vi "sync stream channels.vi"(7 "stream":T1 format="%.0x", 8 "error in":errorcluster, 10 "names":string[](array[string]), 11 "channels":T1[](array[typedef]) format="%.0x") -> (0 "error out":errorcluster, 2 "saved names":string[](array[string]), 3 "saved channels":T1[](array[typedef]) format="%.0x")   [LabVIEW 2026, in "Nominal Core Streaming System Explorer.lvlib"]
uses:
  Nominal Core Streaming System Explorer.lvlib
  <vilib>/NI VeriStand/Custom Device API/Custom Device Item Ref.ctl
  <vilib>/NI VeriStand/Custom Device API/Set Item Property (String Array).vi
  <vilib>/NI VeriStand/Custom Device API/Custom Device API.lvlib
  <vilib>/NI VeriStand/Custom Device Tools/Custom Device Utility Library/Custom Device Utility Library.lvlib
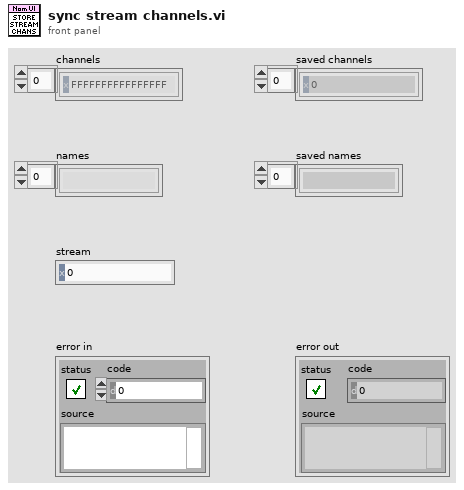
[diagram p1: front panel]
types:
  T1 = typedef "Custom Device API.lvlib/Custom Device Item Ref.ctl" = u64
  T2 = typedef "Custom Device API.lvlib/Custom Device Item Info.ctl" = cluster{"Name":string, "Is Channel":bool, "GUID":string, "Is Waveform":bool}
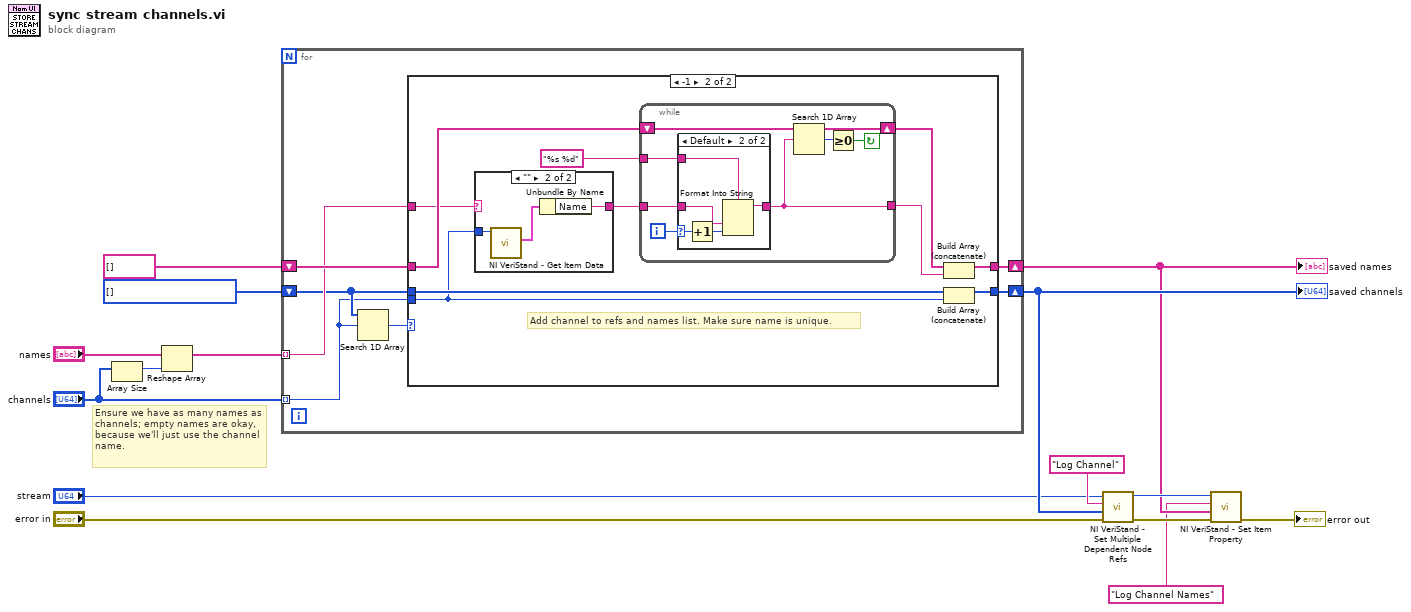
[diagram p0: block diagram]
diagram:
  # "Ensure we have as many names as channels; empty names are okay, because we'll just use the channel name."
  n1 = Array Size(array="channels") -> (size(s)=w5:i32)
  n2 = Reshape Array("names", w5) -> (w6:string[])
  n3 = for {
    shift-right: [w22] -> w15
    shift-left: T1[] [] ("Selected Channel Refs") -> [w18]
    shift-right: [w20] -> w2
    shift-left: string[] [] -> [w21]
    tunnel: "channels" -> [w16] mode=indexing
    tunnel: w6 -> [w19] mode=indexing
    n4 = Search 1D Array(1D array=w18, element=w16) -> (index of element=w17:i32)  [unwired: 1 out]
    n5 = case shown="-1" w17 {
      tunnel: w18 -> [w24 w34]
      tunnel: [w24 w33] -> w22
      tunnel: w16 -> [_ w32]
      tunnel: w21 -> [w23 w28]
      tunnel: [w23 w31] -> w20
      tunnel: w19 -> [_ w25]
      frame Default {
        # "Channel already selected for logging. Don't add to refs or names list."
      }
      frame -1 {
        # "Add channel to refs and names list. Make sure name is unique."
        n6 = case shown="\"\"" w25 {
          selector: w25 -> [w35 _]
          tunnel: w32 -> [_ w38]
          tunnel: [w35 w36] -> w27
          frame Default {
          }
          frame "" {
            n7 = call <vilib>:"NI VeriStand - Get Item Data.vi"("Item Ref in"=w38) -> ("Item Info"=w37:T2)  [unwired: 1 in, 9 out]
            n8 = Unbundle By Name(w37) -> ("Name"=w36:string)
          }
        }
        n9 = while {
          shift-right: [w43] -> w29
          shift-left: w28 -> [w43]
          tunnel: w27 -> [w44]
          tunnel: [w40] -> w26
          tunnel: "%s %d" ("format string") -> [w39]
          i -> [w45]
          stop <- w41 continue-if-true
          n10 = case shown="Default" w45 {
            selector: w45 -> [_ w49]
            tunnel: w44 -> [w46 w47]
            tunnel: [w46 w51] -> w40
            tunnel: w39 -> [_ w50]
            frame 0 {
            }
            frame Default {
              n11 = Increment(x=w49) -> (x+1=w48:i32)
              n12 = Format Into String(format string=w50, w47, w48) -> (resulting string=w51:string)  [unwired: 2 in, 1 out]
            }
          }
          n13 = Search 1D Array(1D array=w43, element=w40) -> (index of element=w42:i32)  [unwired: 1 out]
          n14 = Greater Or Equal To 0?(x=w42) -> (x >= 0?=w41:bool)
        }
        n15 = Build Array (concatenate)(w29, w26) -> (w31:string[])
        n16 = Build Array (concatenate)(w34, w32) -> (w33:T1[])
      }
    }
  }
  "saved channels" <- w15
  "saved names" <- w2
  n17 = call <vilib>:"NI VeriStand - Set Multiple Dependent Node Refs.vi"("error in (no error)"="error in", "Dependent Node Refs"=w15, "Base Property Name"="Log Channel" ("Property Name"), "Item Ref in"="stream") -> ("error out"=w13:errorcluster, "Item Ref out"=w3:T1)  [unwired: 6 in]
  n18 = call-poly <vilib>:"NI VeriStand - Set Item Property.vi"("error in (no error)"=w13, "Value"=w2, "Property Name"="Log Channel Names", "Item Ref in"=w3) -> ("error out"=→"error out":errorcluster)  [unwired: 5 in, 2 out]
